vi "Non equal Min Max.vi"(1 "Start precision":i32, 2 "Max":dbl, 3 "Min":dbl) -> (0 "Limits":string)   [LabVIEW 2022 SP3]
panel:
  out "Range in":dbl
  out "Range out":dbl
  out "Top Limit":string
  out "Bottom Limit":string
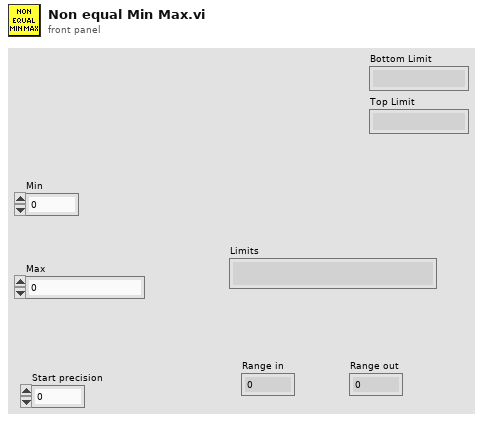
[diagram p1: front panel]
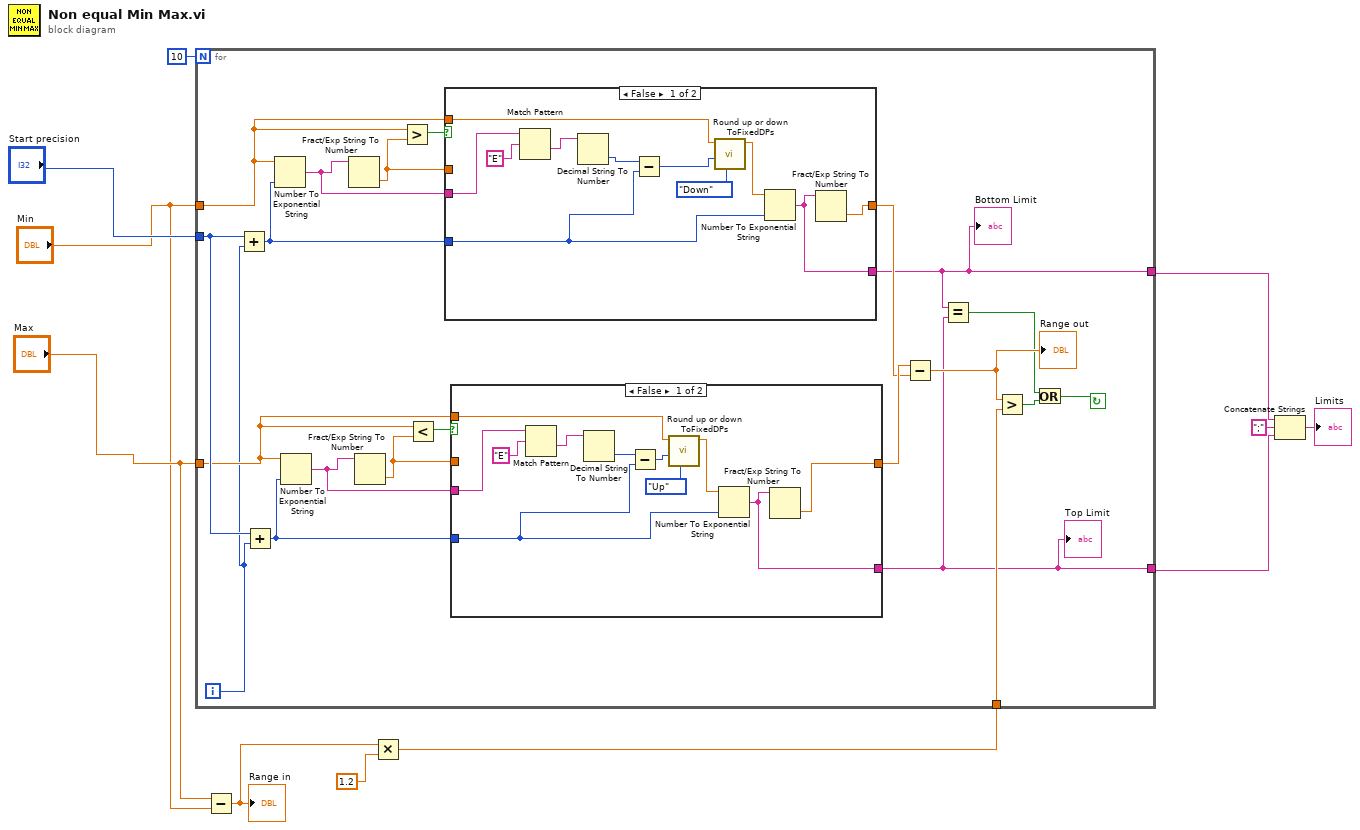
[diagram p0: block diagram]
diagram:
  n1 = Subtract(x="Max", y="Min") -> (x-y=w7:dbl)
  "Range in" <- w7
  n2 = Multiply(x=w7, y=1.2) -> (x*y=w5:dbl)
  n3 = for {
    N: 10 -> [_]
    tunnel: [w13] -> w2
    tunnel: [w12] -> w1
    tunnel: "Start precision" -> [w32]
    tunnel: "Max" -> [w23]
    tunnel: "Min" -> [w22]
    tunnel: w5 -> [w18]
    i -> [w21]
    stop <- w14 continue-if-true
    n4 = Add(x=w32, y=w21) -> (x+y=w29:i32)
    n5 = Add(x=w32, y=w21) -> (x+y=w25:i32)
    n6 = Number To Exponential String(number=w22, precision (6)=w29) -> (E-format string=w30:string)  [unwired: 2 in]
    n7 = Number To Exponential String(number=w23, precision (6)=w25) -> (E-format string=w26:string)  [unwired: 2 in]
    n8 = Fract/Exp String To Number(string=w30) -> (number=w28:dbl)  [unwired: 3 in, 1 out]
    n9 = Fract/Exp String To Number(string=w26) -> (number=w24:dbl)  [unwired: 3 in, 1 out]
    n10 = Greater?(x=w22, y=w28) -> (0:w31:bool)
    n11 = Less?(x=w23, y=w24) -> (x < y?=w27:bool)
    n12 = case shown="False" w31 {
      tunnel: w22 -> [w51 _]
      tunnel: w30 -> [w53 w58]
      tunnel: w29 -> [w46 _]
      tunnel: [w50 w58] -> w13
      tunnel: [w49 w57] -> w19
      tunnel: w28 -> [_ w57]
      frame False {
        n13 = Match Pattern(string=w53, regular expression="E") -> (after substring=w55:string)  [unwired: 1 in, 3 out]
        n14 = Decimal String To Number(string=w55) -> (number=w48:i32)  [unwired: 2 in, 1 out]
        n15 = Subtract(x=w48, y=w46) -> (x-y=w47:i32)
        n16 = call "Round up or down ToFixedDPs.vi"("Round"=enum16{"Up", "Down", "Nearest"}."Down", "Power of ten"=w47, "Number to round"=w51) -> ("Rounded number"=w52:dbl)  [unwired: 7 in, 1 out]
        n17 = Number To Exponential String(number=w52, precision (6)=w46) -> (E-format string=w50:string)  [unwired: 2 in]
        n18 = Fract/Exp String To Number(string=w50) -> (number=w49:dbl)  [unwired: 3 in, 1 out]
      }
      frame True {
      }
    }
    "Bottom Limit" <- w13
    n19 = case shown="False" w27 {
      tunnel: w23 -> [w38 _]
      tunnel: w26 -> [w40 w45]
      tunnel: w25 -> [w33 _]
      tunnel: [w37 w45] -> w12
      tunnel: [w36 w44] -> w20
      tunnel: w24 -> [_ w44]
      frame False {
        n20 = Match Pattern(string=w40, regular expression="E") -> (after substring=w42:string)  [unwired: 1 in, 3 out]
        n21 = Decimal String To Number(string=w42) -> (number=w34:i32)  [unwired: 2 in, 1 out]
        n22 = Subtract(x=w34, y=w33) -> (x-y=w35:i32)
        n23 = call "Round up or down ToFixedDPs.vi"("Round"=enum16{"Up", "Down", "Nearest"}."Up", "Power of ten"=w35, "Number to round"=w38) -> ("Rounded number"=w39:dbl)  [unwired: 7 in, 1 out]
        n24 = Number To Exponential String(number=w39, precision (6)=w33) -> (E-format string=w37:string)  [unwired: 2 in]
        n25 = Fract/Exp String To Number(string=w37) -> (number=w36:dbl)  [unwired: 3 in, 1 out]
      }
      frame True {
      }
    }
    "Top Limit" <- w12
    n26 = Subtract(x=w20, y=w19) -> (x-y=w17:dbl)
    "Range out" <- w17
    n27 = Equal?(x=w13, y=w12) -> (x = y?=w15:bool)
    n28 = Greater?(x=w17, y=w18) -> (0:w16:bool)
    n29 = Or(x=w15, y=w16) -> (x .or. y?=w14:bool)
  }
  n30 = Concatenate Strings(w2, ";" ("string"), w1) -> (→"Limits":string)
